vi "RangeCheck.vi"(0 "NhRegenGridSim in":refnum<class "NHRGridSim.lvclass">, 1 "RangeCheck":T1, 2 "Phase":i32, 3 "error in (no error)":errorcluster) -> (7 "NhRegenGridSim out":refnum<class "NHRGridSim.lvclass">, 10 "error out":errorcluster)   [LabVIEW 2018, in "AcPwrPlugins.lvlib" / "NHRGridSim.lvclass"]
doc: "This VI validates that the properties being set via the prefence dialog or stored in the INI file are valid."
uses:
  NHRGridSim.lvclass
  TypeDefs/RangeCheck.ctl
  <instrlib>/NH Research 9400 Series/Public/Utility/Query Capabilities (Current).vi
  <vilib>/Utility/error.llb/Error Cluster From Error Code.vi
  <instrlib>/NH Research 9400 Series/Public/Utility/Query Capabilities (Voltage).vi
  <instrlib>/NH Research 9400 Series/Public/Utility/Query Capabilities (Power).vi
  <instrlib>/NH Research 9400 Series/Public/Utility/Query Capabilities (Frequency).vi
  <instrlib>/NH Research 9400 Series/Public/Utility/Query Capabilities (Aperture).vi
  <instrlib>/NH Research 9400 Series/Public/Utility/Query Capabilities (Sample).vi
  <instrlib>/NH Research 9400 Series/Public/Utility/Query Capabilities (Phase Angle).vi
  <vilib>/ErrorRing/Error Ring.xnode
  <instrlib>/NH Research 9400 Series/NH Research 9400 Series.lvlib
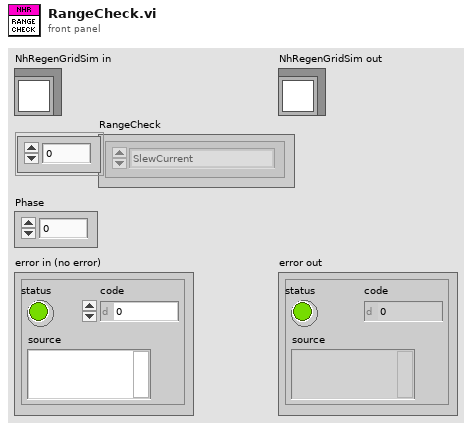
[diagram p1: front panel]
types:
  T1 = typedef "AcPwrPlugins.lvlib/NHRGridSim.lvclass/RangeCheck.ctl" = enum16{"SlewCurrent", "SlewVoltage", "SlewPower", "SlewFrequency", "ApertureLength", "NumberOfSamples", "SlewAngleMultiPhaseAB", "SlewAngleMultiPhaseAC", "VoltageRange", "CurrentRange", "PhaseAngle", "Power", "Current", "Voltage", "Frequency"}[]
  T2 = typedef "AcPwrPlugins.lvlib/NHRGridSim.lvclass/DeviceSettings.ctl" = cluster{"SlewRates":cluster{"Islew":dbl, "Vslew":dbl, "Pslew":dbl, "FreqSlew":dbl, "AngleABSlew":dbl, "AngleACSlew":dbl}, "Phases":cluster{"Pout (W)":dbl, "Iout (A)":dbl, "PhaseAngle":dbl, "Vout (V)":dbl, "Phase Name":string}[], "Measurement":cluster{"ApertureLength (s)":dbl, "NumberOfSamples":u32}, "Ranges":cluster{"Irange (A)":dbl, "Vrange (V)":dbl}, "Mode":enum8{"One 3-Phase AC", "One AC", "One DC", "Three AC", "Three DC", "One 2-Phase AC and One AC", "One 2-Phase AC and One DC", "Two AC", "One AC and One DC", "Two AC and One DC", "One AC and Two DC", "One DC and One AC", "Two DC"}, "PowerMax":u16, "TransformerRatio":dbl, "Waveshape":dbl[], "Handle":string, "FreqOut (Hz)":dbl, "Connected":bool, "Safety Limits":cluster{"Minimum Voltage (V)":dbl, "Minimum Voltage Time (s)":dbl, "Maximum Voltage (V)":dbl, "Maximum Voltage Time (s)":dbl, "Maximum Source Amps (A)":dbl, "Maximum Source Amps Time (s)":dbl, "Maximum Sink Amps (A)":dbl, "Maximum Sink Amps Time (s)":dbl, "Maximum Source Power (W)":dbl, "Maximum Source Power Time (s)":dbl, "Maximum Sink Power (W)":dbl, "Maximum Sink Power Time (s)":dbl, "Peak Voltage (V)":dbl, "Peak Voltage Enable":bool, "Peak Amps (A)":dbl, "Peak Amps Enable":bool}, "btnIdQuery":bool, "btnReset":bool, "Initialize Timeout (10000 ms)":u32}[]
  T3 = typedef "NH Research 9400 Series.lvlib/Current Capabilities.ctl" = cluster{"Module Min (A)":dbl, "Module Max (A)":dbl, "Range Min (A)":dbl, "Range Max (A)":dbl, "Measure Min (A)":dbl, "Measure Max (A)":dbl, "Measure Range Min (A)":dbl, "Measure Range Max (A)":dbl, "Slew Min (A per sec)":dbl, "Slew Max (A per sec)":dbl, "Slew Range Min (A per sec)":dbl, "Slew Range Max (A per sec)":dbl}
  T4 = typedef "NH Research 9400 Series.lvlib/Voltage Capabilities.ctl" = cluster{"Module Min (V)":dbl, "Module Max (V)":dbl, "Range Min (V)":dbl, "Range Max (V)":dbl, "Measure Min (V)":dbl, "Measure Max (V)":dbl, "Measure Range Min (V)":dbl, "Measure Range Max (V)":dbl, "Slew Min (V per sec)":dbl, "Slew Max (V per sec)":dbl, "Slew Range Min (V per sec)":dbl, "Slew Range Max (V per sec)":dbl}
  T5 = typedef "NH Research 9400 Series.lvlib/Power Capabilities.ctl" = cluster{"Module Min (W)":dbl, "Module Max (W)":dbl, "Range Min (W)":dbl, "Range Max (W)":dbl, "Slew Min (W per sec)":dbl, "Slew Max (W per sec)":dbl, "Slew Range Min (W per sec)":dbl, "Slew Range Max (W per sec)":dbl}
  T6 = typedef "NH Research 9400 Series.lvlib/Frequency Capabilities.ctl" = cluster{"Module Min (Hz)":dbl, "Module Max (Hz)":dbl, "Range Min (Hz)":dbl, "Range Max (Hz)":dbl, "Slew Min (Hz per sec)":dbl, "Slew Max (Hz per sec)":dbl, "Slew Range Min (Hz per sec)":dbl, "Slew Range Max (Hz per sec)":dbl}
  T7 = typedef "NH Research 9400 Series.lvlib/Phase Capabilities.ctl" = cluster{"Slew Min (deg per sec)":dbl, "Slew Max (deg per sec)":dbl, "Slew Range Min (deg per sec)":dbl, "Slew Range Max (deg per sec)":dbl}
  T8 = cluster{"Pout (W)":dbl, "Iout (A)":dbl, "PhaseAngle":dbl, "Vout (V)":dbl, "Phase Name":string}[]
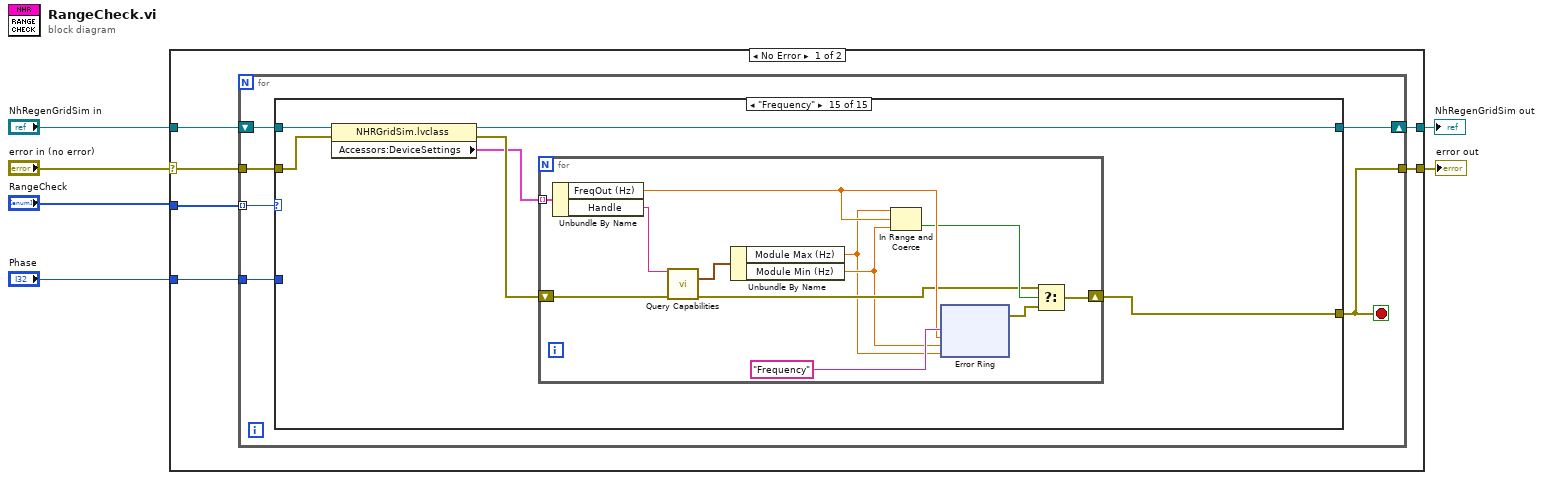
[diagram p0: block diagram]
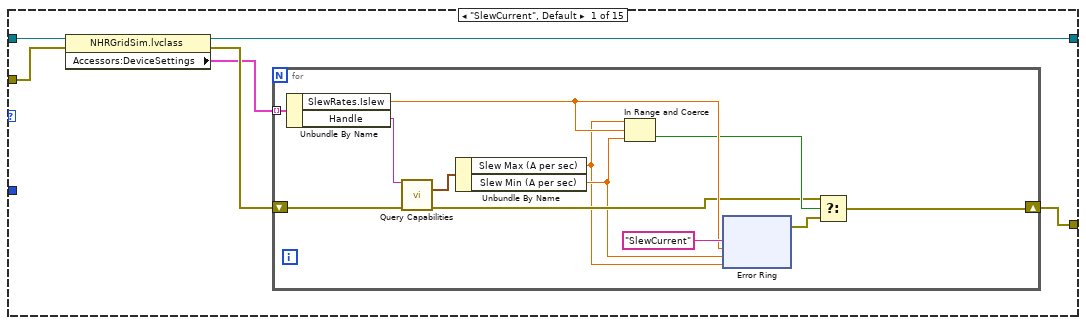
[diagram p2: hidden frame]
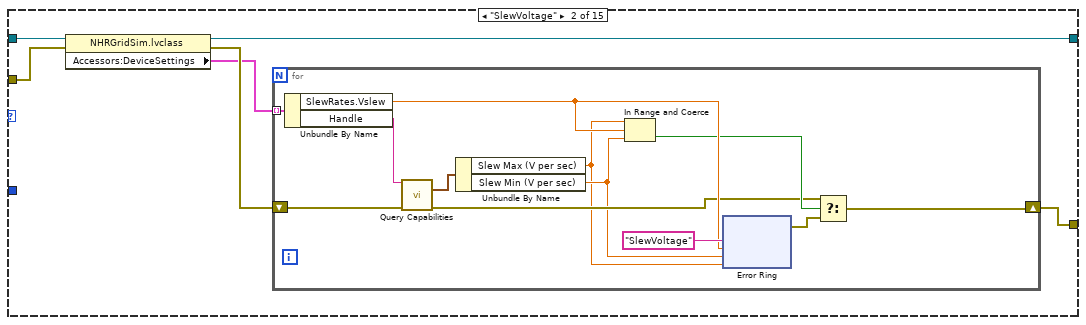
[diagram p3: hidden frame]
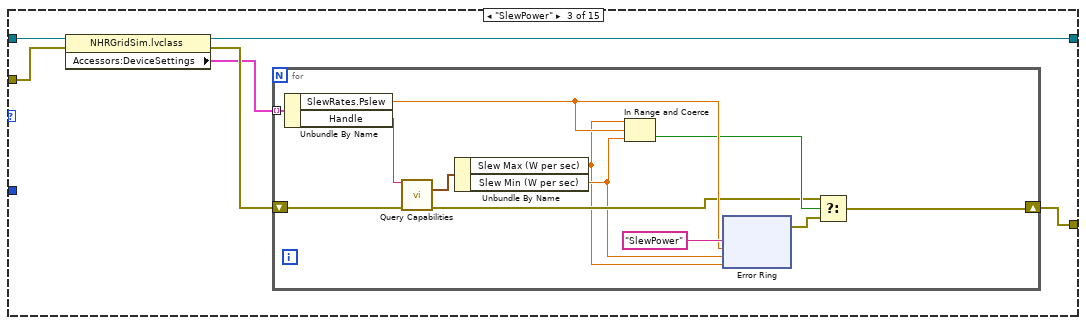
[diagram p4: hidden frame]
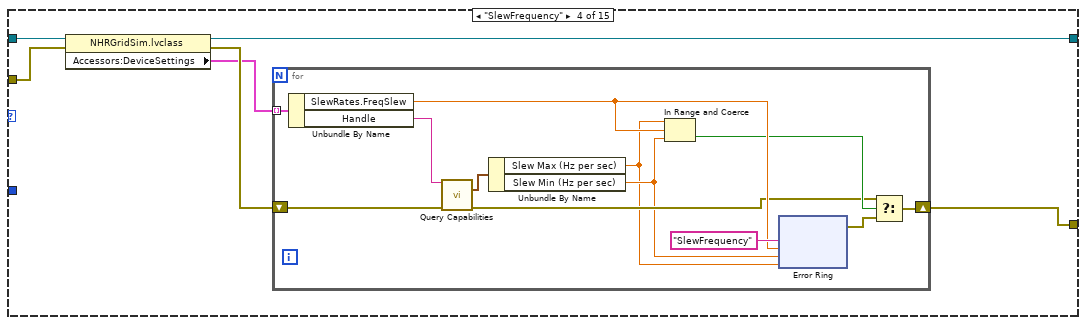
[diagram p5: hidden frame]
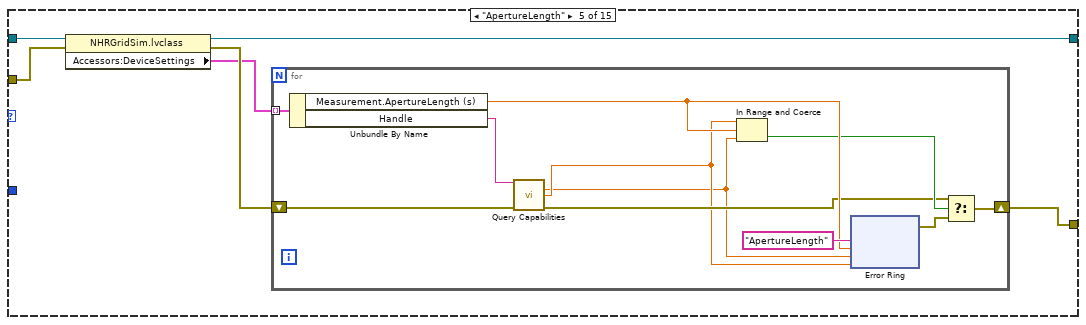
[diagram p6: hidden frame]
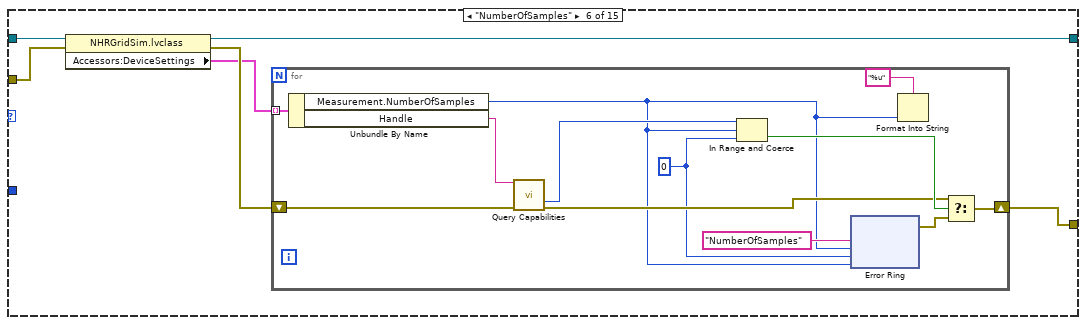
[diagram p7: hidden frame]
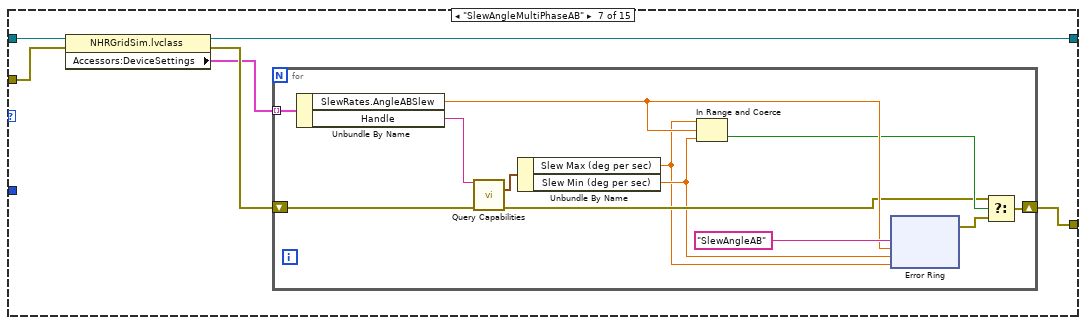
[diagram p8: hidden frame]
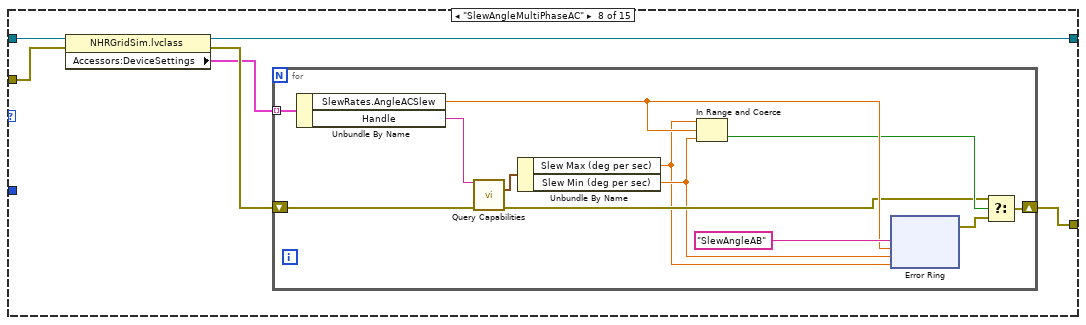
[diagram p9: hidden frame]
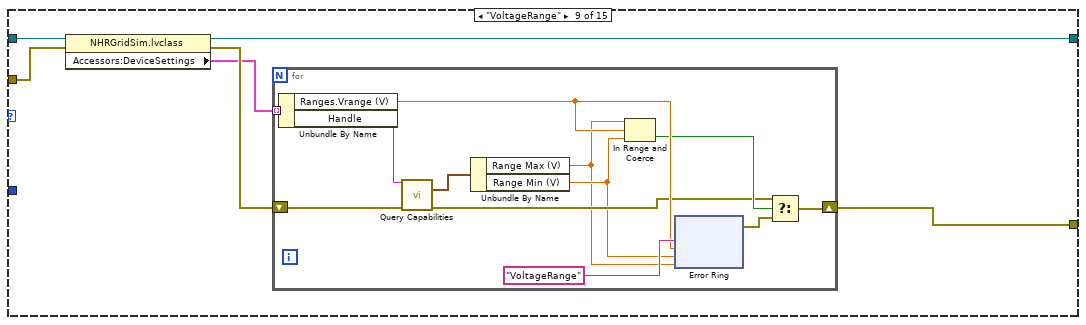
[diagram p10: hidden frame]
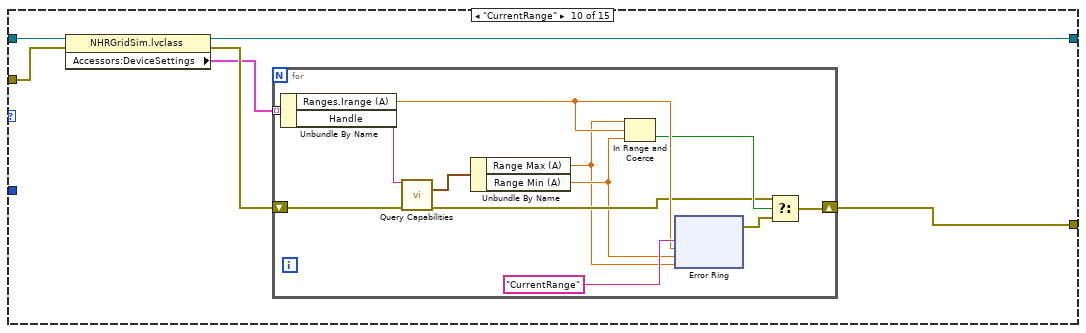
[diagram p11: hidden frame]
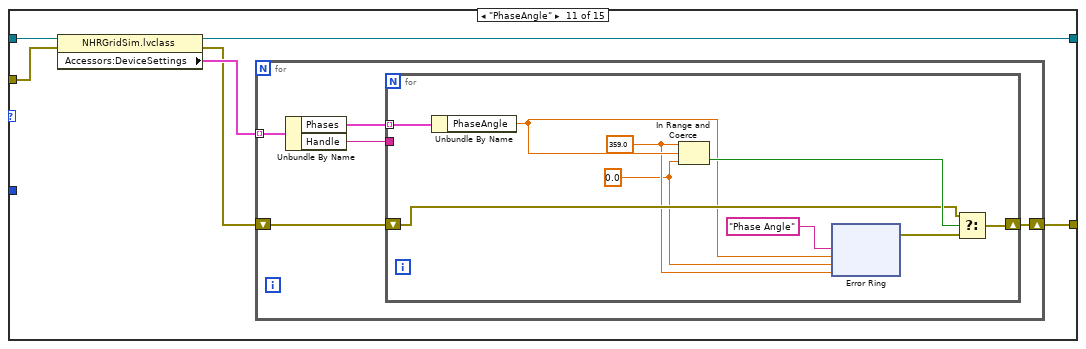
[diagram p12: hidden frame]
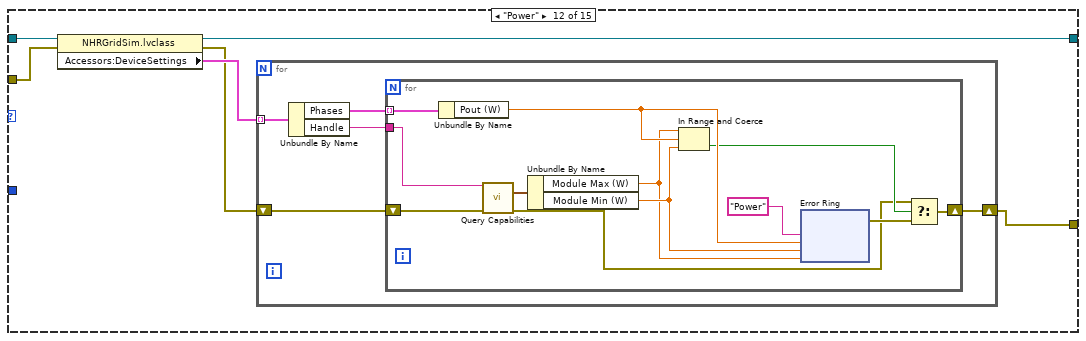
[diagram p13: hidden frame]
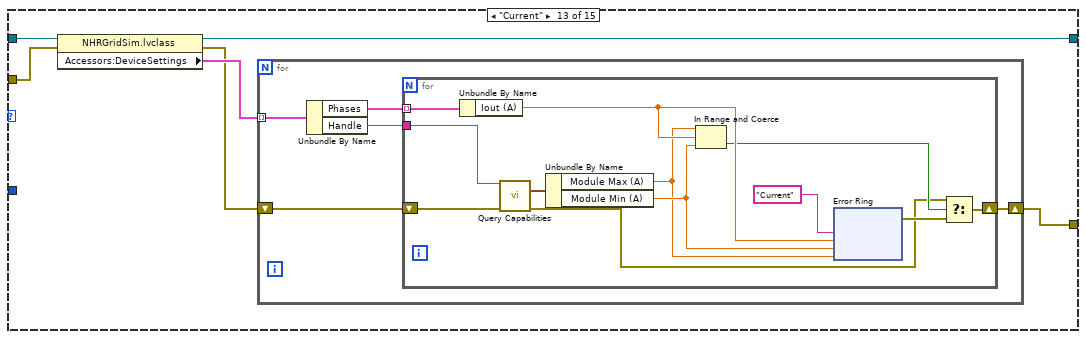
[diagram p14: hidden frame]
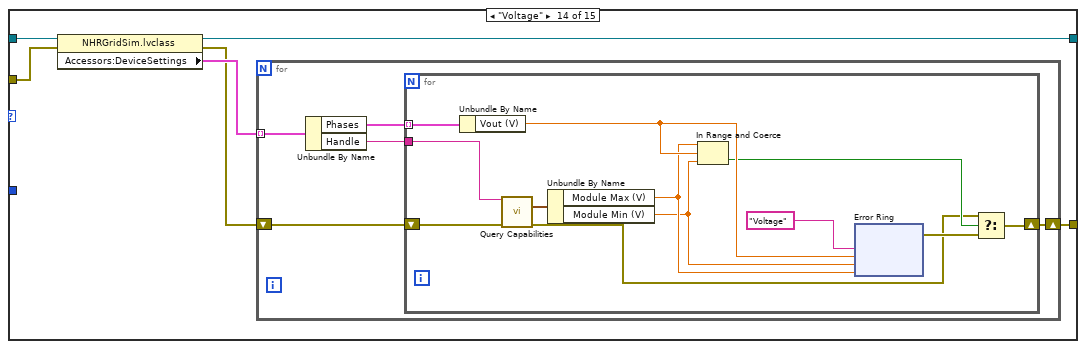
[diagram p15: hidden frame]
diagram:
  n1 = case shown="No Error" "error in (no error)" {
    selector: "error in (no error)" -> [w12 w453]
    tunnel: "Phase" -> [w11 _]
    tunnel: "NhRegenGridSim in" -> [w10 w454]
    tunnel: [w9 w454] -> w3
    tunnel: [w8 w453] -> w2
    tunnel: "RangeCheck" -> [w7 _]
    frame No Error {
      n2 = for {
        tunnel: w7 -> [w18] mode=indexing
        tunnel: w11 -> [w16]
        shift-right: [w15] -> w9
        shift-left: w10 -> [w17]
        tunnel: [w14] -> w8
        tunnel: w12 -> [w13]
        stop <- w14 stop-if-true
        n3 = case shown="\"Frequency\"" w18 {
          tunnel: w17 -> [w24 w52 w80 w108 w136 w163 w191 w219 w247 w275 w303 w333 w366 w397 w430]
          tunnel: w16 -> [_ _ _ _ _ _ _ _ _ _ _ _ _ _ _]
          tunnel: [w23 w51 w79 w107 w135 w162 w190 w218 w246 w274 w302 w332 w365 w396 w429] -> w15
          tunnel: [w21 w49 w77 w105 w133 w160 w188 w216 w244 w272 w299 w329 w362 w393 w427] -> w14
          tunnel: w13 -> [w20 w48 w76 w104 w132 w159 w187 w215 w243 w271 w298 w328 w361 w392 w426]
          frame "SlewCurrent", Default {
            n4 = property class="NHRGridSim.lvclass"(reference=w24, error in=w20) -> (reference out=w23:refnum<class "NHRGridSim.lvclass">, error out=w22:errorcluster, "Accessors:DeviceSettings"=w19:T2)
            n5 = for {
              tunnel: w19 -> [w33] mode=indexing
              shift-right: [w34] -> w21
              shift-left: w22 -> [w31]
              n6 = Unbundle By Name(w33) -> ("SlewRates.Islew"=w29:dbl, "Handle"=w32:string)
              n7 = call-poly <instrlib>:"Query Capabilities.vi"("VISA resource name"=w32, "error in (no error)"=w31) -> ("Current Capabilities"=w30:T3, "error out"=w27:errorcluster)  [unwired: 11 in, 1 out]
              n8 = Unbundle By Name(w30) -> ("Slew Max (A per sec)"=w25:dbl, "Slew Min (A per sec)"=w26:dbl)
              n9 = In Range and Coerce(upper limit=w25, x=w29, lower limit=w26) -> (In Range?=w28:bool)  [unwired: 1 out]
              n10 = xnode "Error Ring"("parameter 0"="SlewCurrent", "parameter 1"=w29, "parameter 2"=w26, "parameter 3"=w25) -> ("error out"=w35:errorcluster)
              n11 = Select(t=w27, s=w28, f=w35) -> (s? t:f=w34:errorcluster)
            }
          }
          frame "SlewVoltage" {
            n12 = property class="NHRGridSim.lvclass"(reference=w52, error in=w48) -> (reference out=w51:refnum<class "NHRGridSim.lvclass">, error out=w50:errorcluster, "Accessors:DeviceSettings"=w47:T2)
            n13 = for {
              tunnel: w47 -> [w61] mode=indexing
              shift-right: [w62] -> w49
              shift-left: w50 -> [w59]
              n14 = Unbundle By Name(w61) -> ("SlewRates.Vslew"=w57:dbl, "Handle"=w60:string)
              n15 = call-poly <instrlib>:"Query Capabilities.vi"("VISA resource name"=w60, "error in (no error)"=w59) -> ("Voltage Capabilities"=w58:T4, "error out"=w55:errorcluster)  [unwired: 11 in, 1 out]
              n16 = Unbundle By Name(w58) -> ("Slew Max (V per sec)"=w53:dbl, "Slew Min (V per sec)"=w54:dbl)
              n17 = In Range and Coerce(upper limit=w53, x=w57, lower limit=w54) -> (In Range?=w56:bool)  [unwired: 1 out]
              n18 = xnode "Error Ring"("parameter 0"="SlewVoltage", "parameter 1"=w57, "parameter 2"=w54, "parameter 3"=w53) -> ("error out"=w63:errorcluster)
              n19 = Select(t=w55, s=w56, f=w63) -> (s? t:f=w62:errorcluster)
            }
          }
          frame "SlewPower" {
            n20 = property class="NHRGridSim.lvclass"(reference=w80, error in=w76) -> (reference out=w79:refnum<class "NHRGridSim.lvclass">, error out=w78:errorcluster, "Accessors:DeviceSettings"=w75:T2)
            n21 = for {
              tunnel: w75 -> [w89] mode=indexing
              shift-right: [w90] -> w77
              shift-left: w78 -> [w87]
              n22 = Unbundle By Name(w89) -> ("SlewRates.Pslew"=w85:dbl, "Handle"=w88:string)
              n23 = call-poly <instrlib>:"Query Capabilities.vi"("VISA resource name"=w88, "error in (no error)"=w87) -> ("Power Capabilities"=w86:T5, "error out"=w83:errorcluster)  [unwired: 11 in, 1 out]
              n24 = Unbundle By Name(w86) -> ("Slew Max (W per sec)"=w81:dbl, "Slew Min (W per sec)"=w82:dbl)
              n25 = In Range and Coerce(upper limit=w81, x=w85, lower limit=w82) -> (In Range?=w84:bool)  [unwired: 1 out]
              n26 = xnode "Error Ring"("parameter 0"="SlewPower", "parameter 1"=w85, "parameter 2"=w82, "parameter 3"=w81) -> ("error out"=w91:errorcluster)
              n27 = Select(t=w83, s=w84, f=w91) -> (s? t:f=w90:errorcluster)
            }
          }
          frame "SlewFrequency" {
            n28 = property class="NHRGridSim.lvclass"(reference=w108, error in=w104) -> (reference out=w107:refnum<class "NHRGridSim.lvclass">, error out=w106:errorcluster, "Accessors:DeviceSettings"=w103:T2)
            n29 = for {
              tunnel: w103 -> [w117] mode=indexing
              shift-right: [w118] -> w105
              shift-left: w106 -> [w115]
              n30 = Unbundle By Name(w117) -> ("SlewRates.FreqSlew"=w113:dbl, "Handle"=w116:string)
              n31 = call-poly <instrlib>:"Query Capabilities.vi"("VISA resource name"=w116, "error in (no error)"=w115) -> ("Frequency Capabilities"=w114:T6, "error out"=w111:errorcluster)  [unwired: 11 in, 1 out]
              n32 = Unbundle By Name(w114) -> ("Slew Max (Hz per sec)"=w109:dbl, "Slew Min (Hz per sec)"=w110:dbl)
              n33 = In Range and Coerce(upper limit=w109, x=w113, lower limit=w110) -> (In Range?=w112:bool)  [unwired: 1 out]
              n34 = xnode "Error Ring"("parameter 0"="SlewFrequency", "parameter 1"=w113, "parameter 2"=w110, "parameter 3"=w109) -> ("error out"=w119:errorcluster)
              n35 = Select(t=w111, s=w112, f=w119) -> (s? t:f=w118:errorcluster)
            }
          }
          frame "ApertureLength" {
            n36 = property class="NHRGridSim.lvclass"(reference=w136, error in=w132) -> (reference out=w135:refnum<class "NHRGridSim.lvclass">, error out=w134:errorcluster, "Accessors:DeviceSettings"=w131:T2)
            n37 = for {
              tunnel: w131 -> [w144] mode=indexing
              shift-right: [w145] -> w133
              shift-left: w134 -> [w142]
              n38 = Unbundle By Name(w144) -> ("Measurement.ApertureLength (s)"=w141:dbl, "Handle"=w143:string)
              n39 = call-poly <instrlib>:"Query Capabilities.vi"("VISA resource name"=w143, "error in (no error)"=w142) -> ("Aperture Min (s)"=w137:dbl, "Aperture Max (s)"=w138:dbl, "error out"=w139:errorcluster)  [unwired: 10 in, 1 out]
              n40 = In Range and Coerce(upper limit=w138, x=w141, lower limit=w137) -> (In Range?=w140:bool)  [unwired: 1 out]
              n41 = xnode "Error Ring"("parameter 0"="ApertureLength", "parameter 1"=w141, "parameter 2"=w137, "parameter 3"=w138) -> ("error out"=w146:errorcluster)
              n42 = Select(t=w139, s=w140, f=w146) -> (s? t:f=w145:errorcluster)
            }
          }
          frame "NumberOfSamples" {
            n43 = property class="NHRGridSim.lvclass"(reference=w163, error in=w159) -> (reference out=w162:refnum<class "NHRGridSim.lvclass">, error out=w161:errorcluster, "Accessors:DeviceSettings"=w158:T2)
            n44 = for {
              tunnel: w158 -> [w172] mode=indexing
              shift-right: [w173] -> w160
              shift-left: w161 -> [w170]
              w165 = u32 0 ("lower limit")
              n45 = Unbundle By Name(w172) -> ("Measurement.NumberOfSamples"=w164:u32, "Handle"=w171:string)
              n46 = call-poly <instrlib>:"Query Capabilities.vi"("VISA resource name"=w171, "error in (no error)"=w170) -> ("Points"=w167:u32, "error out"=w168:errorcluster)  [unwired: 9 in, 3 out]
              n47 = In Range and Coerce(upper limit=w167, x=w164, lower limit=w165) -> (In Range?=w169:bool)  [unwired: 1 out]
              n48 = xnode "Error Ring"("parameter 0"="NumberOfSamples", "parameter 1"=w164, "parameter 2"=w165, "parameter 3"=w164) -> ("error out"=w174:errorcluster)
              n49 = Format Into String(format string="%u", w164) -> ()  [unwired: 2 in, 2 out]
              n50 = Select(t=w168, s=w169, f=w174) -> (s? t:f=w173:errorcluster)
            }
          }
          frame "SlewAngleMultiPhaseAB" {
            n51 = property class="NHRGridSim.lvclass"(reference=w191, error in=w187) -> (reference out=w190:refnum<class "NHRGridSim.lvclass">, error out=w189:errorcluster, "Accessors:DeviceSettings"=w186:T2)
            n52 = for {
              tunnel: w186 -> [w200] mode=indexing
              shift-right: [w201] -> w188
              shift-left: w189 -> [w198]
              n53 = Unbundle By Name(w200) -> ("SlewRates.AngleABSlew"=w196:dbl, "Handle"=w199:string)
              n54 = call-poly <instrlib>:"Query Capabilities.vi"("VISA resource name"=w199, "error in (no error)"=w198) -> ("Phase Angle Capabilities"=w197:T7, "error out"=w194:errorcluster)  [unwired: 11 in, 1 out]
              n55 = Unbundle By Name(w197) -> ("Slew Max (deg per sec)"=w192:dbl, "Slew Min (deg per sec)"=w193:dbl)
              n56 = In Range and Coerce(upper limit=w192, x=w196, lower limit=w193) -> (In Range?=w195:bool)  [unwired: 1 out]
              n57 = xnode "Error Ring"("parameter 0"="SlewAngleAB", "parameter 1"=w196, "parameter 2"=w193, "parameter 3"=w192) -> ("error out"=w202:errorcluster)
              n58 = Select(t=w194, s=w195, f=w202) -> (s? t:f=w201:errorcluster)
            }
          }
          frame "SlewAngleMultiPhaseAC" {
            n59 = property class="NHRGridSim.lvclass"(reference=w219, error in=w215) -> (reference out=w218:refnum<class "NHRGridSim.lvclass">, error out=w217:errorcluster, "Accessors:DeviceSettings"=w214:T2)
            n60 = for {
              tunnel: w214 -> [w228] mode=indexing
              shift-right: [w229] -> w216
              shift-left: w217 -> [w226]
              n61 = Unbundle By Name(w228) -> ("SlewRates.AngleACSlew"=w224:dbl, "Handle"=w227:string)
              n62 = call-poly <instrlib>:"Query Capabilities.vi"("VISA resource name"=w227, "error in (no error)"=w226) -> ("Phase Angle Capabilities"=w225:T7, "error out"=w222:errorcluster)  [unwired: 11 in, 1 out]
              n63 = Unbundle By Name(w225) -> ("Slew Max (deg per sec)"=w220:dbl, "Slew Min (deg per sec)"=w221:dbl)
              n64 = In Range and Coerce(upper limit=w220, x=w224, lower limit=w221) -> (In Range?=w223:bool)  [unwired: 1 out]
              n65 = xnode "Error Ring"("parameter 0"="SlewAngleAB", "parameter 1"=w224, "parameter 2"=w221, "parameter 3"=w220) -> ("error out"=w230:errorcluster)
              n66 = Select(t=w222, s=w223, f=w230) -> (s? t:f=w229:errorcluster)
            }
          }
          frame "VoltageRange" {
            n67 = property class="NHRGridSim.lvclass"(reference=w247, error in=w243) -> (reference out=w246:refnum<class "NHRGridSim.lvclass">, error out=w245:errorcluster, "Accessors:DeviceSettings"=w242:T2)
            n68 = for {
              tunnel: w242 -> [w256] mode=indexing
              shift-right: [w257] -> w244
              shift-left: w245 -> [w254]
              n69 = Unbundle By Name(w256) -> ("Ranges.Vrange (V)"=w252:dbl, "Handle"=w255:string)
              n70 = call-poly <instrlib>:"Query Capabilities.vi"("VISA resource name"=w255, "error in (no error)"=w254) -> ("Voltage Capabilities"=w253:T4, "error out"=w250:errorcluster)  [unwired: 11 in, 1 out]
              n71 = Unbundle By Name(w253) -> ("Range Max (V)"=w248:dbl, "Range Min (V)"=w249:dbl)
              n72 = In Range and Coerce(upper limit=w248, x=w252, lower limit=w249) -> (In Range?=w251:bool)  [unwired: 1 out]
              n73 = xnode "Error Ring"("parameter 0"="VoltageRange", "parameter 1"=w252, "parameter 2"=w249, "parameter 3"=w248) -> ("error out"=w258:errorcluster)
              n74 = Select(t=w250, s=w251, f=w258) -> (s? t:f=w257:errorcluster)
            }
          }
          frame "CurrentRange" {
            n75 = property class="NHRGridSim.lvclass"(reference=w275, error in=w271) -> (reference out=w274:refnum<class "NHRGridSim.lvclass">, error out=w273:errorcluster, "Accessors:DeviceSettings"=w270:T2)
            n76 = for {
              tunnel: w270 -> [w284] mode=indexing
              shift-right: [w285] -> w272
              shift-left: w273 -> [w282]
              n77 = Unbundle By Name(w284) -> ("Ranges.Irange (A)"=w280:dbl, "Handle"=w283:string)
              n78 = call-poly <instrlib>:"Query Capabilities.vi"("VISA resource name"=w283, "error in (no error)"=w282) -> ("Current Capabilities"=w281:T3, "error out"=w278:errorcluster)  [unwired: 11 in, 1 out]
              n79 = Unbundle By Name(w281) -> ("Range Max (A)"=w276:dbl, "Range Min (A)"=w277:dbl)
              n80 = In Range and Coerce(upper limit=w276, x=w280, lower limit=w277) -> (In Range?=w279:bool)  [unwired: 1 out]
              n81 = xnode "Error Ring"("parameter 0"="CurrentRange", "parameter 1"=w280, "parameter 2"=w277, "parameter 3"=w276) -> ("error out"=w286:errorcluster)
              n82 = Select(t=w278, s=w279, f=w286) -> (s? t:f=w285:errorcluster)
            }
          }
          frame "PhaseAngle" {
            n83 = property class="NHRGridSim.lvclass"(reference=w303, error in=w298) -> (reference out=w302:refnum<class "NHRGridSim.lvclass">, error out=w300:errorcluster, "Accessors:DeviceSettings"=w301:T2)
            n84 = for {
              tunnel: w301 -> [w306] mode=indexing
              shift-right: [w307] -> w299
              shift-left: w300 -> [w308]
              n85 = Unbundle By Name(w306) -> ("Phases"=w305:T8, "Handle"=w304:string)
              n86 = for {
                shift-right: [w315] -> w307
                shift-left: w308 -> [w312]
                tunnel: w305 -> [w314] mode=indexing
                tunnel: w304 -> [_]
                w310 = 359.0 ("Slew Max (deg per sec)")
                w309 = 0.0 ("Slew Max (deg per sec)")
                n87 = Unbundle By Name(w314) -> ("PhaseAngle"=w311:dbl)
                n88 = In Range and Coerce(upper limit=w310, x=w311, lower limit=w309) -> (In Range?=w313:bool)  [unwired: 1 out]
                n89 = xnode "Error Ring"("parameter 0"="Phase Angle", "parameter 1"=w311, "parameter 2"=w309, "parameter 3"=w310) -> ("error out"=w316:errorcluster)
                n90 = Select(t=w312, s=w313, f=w316) -> (s? t:f=w315:errorcluster)
              }
            }
          }
          frame "Power" {
            n91 = property class="NHRGridSim.lvclass"(reference=w333, error in=w328) -> (reference out=w332:refnum<class "NHRGridSim.lvclass">, error out=w330:errorcluster, "Accessors:DeviceSettings"=w331:T2)
            n92 = for {
              tunnel: w331 -> [w336] mode=indexing
              shift-right: [w337] -> w329
              shift-left: w330 -> [w338]
              n93 = Unbundle By Name(w336) -> ("Phases"=w335:T8, "Handle"=w334:string)
              n94 = for {
                shift-right: [w348] -> w337
                shift-left: w338 -> [w343]
                tunnel: w335 -> [w347] mode=indexing
                tunnel: w334 -> [w342]
                n95 = Unbundle By Name(w347) -> ("Pout (W)"=w346:dbl)
                n96 = call-poly <instrlib>:"Query Capabilities.vi"("VISA resource name"=w342, "error in (no error)"=w343) -> ("Power Capabilities"=w344:T5, "error out"=w341:errorcluster)  [unwired: 11 in, 1 out]
                n97 = Unbundle By Name(w344) -> ("Module Max (W)"=w339:dbl, "Module Min (W)"=w340:dbl)
                n98 = In Range and Coerce(upper limit=w339, x=w346, lower limit=w340) -> (In Range?=w345:bool)  [unwired: 1 out]
                n99 = xnode "Error Ring"("parameter 0"="Power", "parameter 1"=w346, "parameter 2"=w340, "parameter 3"=w339) -> ("error out"=w349:errorcluster)
                n100 = Select(t=w341, s=w345, f=w349) -> (s? t:f=w348:errorcluster)
              }
            }
          }
          frame "Current" {
            n101 = property class="NHRGridSim.lvclass"(reference=w366, error in=w361) -> (reference out=w365:refnum<class "NHRGridSim.lvclass">, error out=w363:errorcluster, "Accessors:DeviceSettings"=w364:T2)
            n102 = for {
              tunnel: w364 -> [w369] mode=indexing
              shift-right: [w370] -> w362
              shift-left: w363 -> [w371]
              n103 = Unbundle By Name(w369) -> ("Phases"=w368:T8, "Handle"=w367:string)
              n104 = for {
                shift-right: [w381] -> w370
                shift-left: w371 -> [w376]
                tunnel: w368 -> [w380] mode=indexing
                tunnel: w367 -> [w375]
                n105 = Unbundle By Name(w380) -> ("Iout (A)"=w379:dbl)
                n106 = call-poly <instrlib>:"Query Capabilities.vi"("VISA resource name"=w375, "error in (no error)"=w376) -> ("Current Capabilities"=w377:T3, "error out"=w374:errorcluster)  [unwired: 11 in, 1 out]
                n107 = Unbundle By Name(w377) -> ("Module Max (A)"=w372:dbl, "Module Min (A)"=w373:dbl)
                n108 = In Range and Coerce(upper limit=w372, x=w379, lower limit=w373) -> (In Range?=w378:bool)  [unwired: 1 out]
                n109 = xnode "Error Ring"("parameter 0"="Current", "parameter 1"=w379, "parameter 2"=w373, "parameter 3"=w372) -> ("error out"=w382:errorcluster)
                n110 = Select(t=w374, s=w378, f=w382) -> (s? t:f=w381:errorcluster)
              }
            }
          }
          frame "Voltage" {
            n111 = property class="NHRGridSim.lvclass"(reference=w397, error in=w392) -> (reference out=w396:refnum<class "NHRGridSim.lvclass">, error out=w394:errorcluster, "Accessors:DeviceSettings"=w395:T2)
            n112 = for {
              tunnel: w395 -> [w400] mode=indexing
              shift-right: [w401] -> w393
              shift-left: w394 -> [w402]
              n113 = Unbundle By Name(w400) -> ("Phases"=w399:T8, "Handle"=w398:string)
              n114 = for {
                shift-right: [w412] -> w401
                shift-left: w402 -> [w407]
                tunnel: w399 -> [w411] mode=indexing
                tunnel: w398 -> [w406]
                n115 = Unbundle By Name(w411) -> ("Vout (V)"=w410:dbl)
                n116 = call-poly <instrlib>:"Query Capabilities.vi"("VISA resource name"=w406, "error in (no error)"=w407) -> ("Voltage Capabilities"=w408:T4, "error out"=w405:errorcluster)  [unwired: 11 in, 1 out]
                n117 = Unbundle By Name(w408) -> ("Module Max (V)"=w404:dbl, "Module Min (V)"=w403:dbl)
                n118 = In Range and Coerce(upper limit=w404, x=w410, lower limit=w403) -> (In Range?=w409:bool)  [unwired: 1 out]
                n119 = xnode "Error Ring"("parameter 0"="Voltage", "parameter 1"=w410, "parameter 2"=w403, "parameter 3"=w404) -> ("error out"=w413:errorcluster)
                n120 = Select(t=w405, s=w409, f=w413) -> (s? t:f=w412:errorcluster)
              }
            }
          }
          frame "Frequency" {
            n121 = property class="NHRGridSim.lvclass"(reference=w430, error in=w426) -> (reference out=w429:refnum<class "NHRGridSim.lvclass">, error out=w428:errorcluster, "Accessors:DeviceSettings"=w425:T2)
            n122 = for {
              tunnel: w425 -> [w439] mode=indexing
              shift-right: [w440] -> w427
              shift-left: w428 -> [w437]
              n123 = Unbundle By Name(w439) -> ("FreqOut (Hz)"=w435:dbl, "Handle"=w438:string)
              n124 = call-poly <instrlib>:"Query Capabilities.vi"("VISA resource name"=w438, "error in (no error)"=w437) -> ("Frequency Capabilities"=w436:T6, "error out"=w433:errorcluster)  [unwired: 11 in, 1 out]
              n125 = Unbundle By Name(w436) -> ("Module Max (Hz)"=w431:dbl, "Module Min (Hz)"=w432:dbl)
              n126 = In Range and Coerce(upper limit=w431, x=w435, lower limit=w432) -> (In Range?=w434:bool)  [unwired: 1 out]
              n127 = xnode "Error Ring"("parameter 0"="Frequency", "parameter 1"=w435, "parameter 2"=w432, "parameter 3"=w431) -> ("error out"=w441:errorcluster)
              n128 = Select(t=w433, s=w434, f=w441) -> (s? t:f=w440:errorcluster)
            }
          }
        }
      }
    }
    frame Error {
    }
  }
  "NhRegenGridSim out" <- w3
  "error out" <- w2
